vi "SetOIDNumbers.vi"(8 "error in (no error)":errorcluster, 11 "RoomAlert in":refnum<class "RoomAlert.lvclass">) -> (0 "error out":errorcluster, 3 "RoomAlert out":refnum<class "RoomAlert.lvclass">)   [LabVIEW 2018, in "SensorPlugins.lvlib" / "RoomAlert.lvclass"]
doc: "Sets the Sensor and the Light Tower OID Numbers that the operator may select from. The Module ID must be correct inorder for this function to work properly thus call GET&SET Instrument information before calling this VI."
uses:
  RoomAlert.lvclass
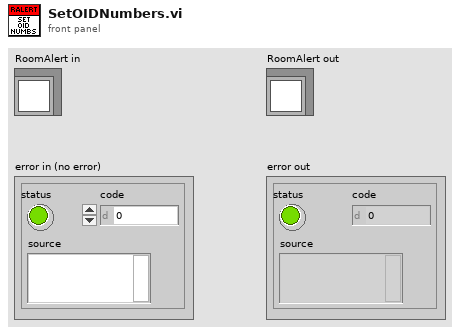
[diagram p1: front panel]
types:
  T1 = typedef "SensorPlugins.lvlib/RoomAlert.lvclass/RoomAlertControls.ctl" = cluster{"Connected?":bool, "IP Address of SNMP Device":string, "Port (161)":u16, "Community Name":string, "Measurements To Read Array":u16[], "Update LightTower?":bool, "LightTower":cluster{"Red":bool, "Amber":bool, "Green":bool, "Audio":bool}, "RoomAlert Model ID":string, "Sensor OID Numbers":string[][], "Sensor Light Tower OID Numbers":string[][]}[]
  T2 = cluster{"Connected?":bool, "IP Address of SNMP Device":string, "Port (161)":u16, "Community Name":string, "Measurements To Read Array":u16[], "Update LightTower?":bool, "LightTower":cluster{"Red":bool, "Amber":bool, "Green":bool, "Audio":bool}, "RoomAlert Model ID":string, "Sensor OID Numbers":string[][], "Sensor Light Tower OID Numbers":string[][]}
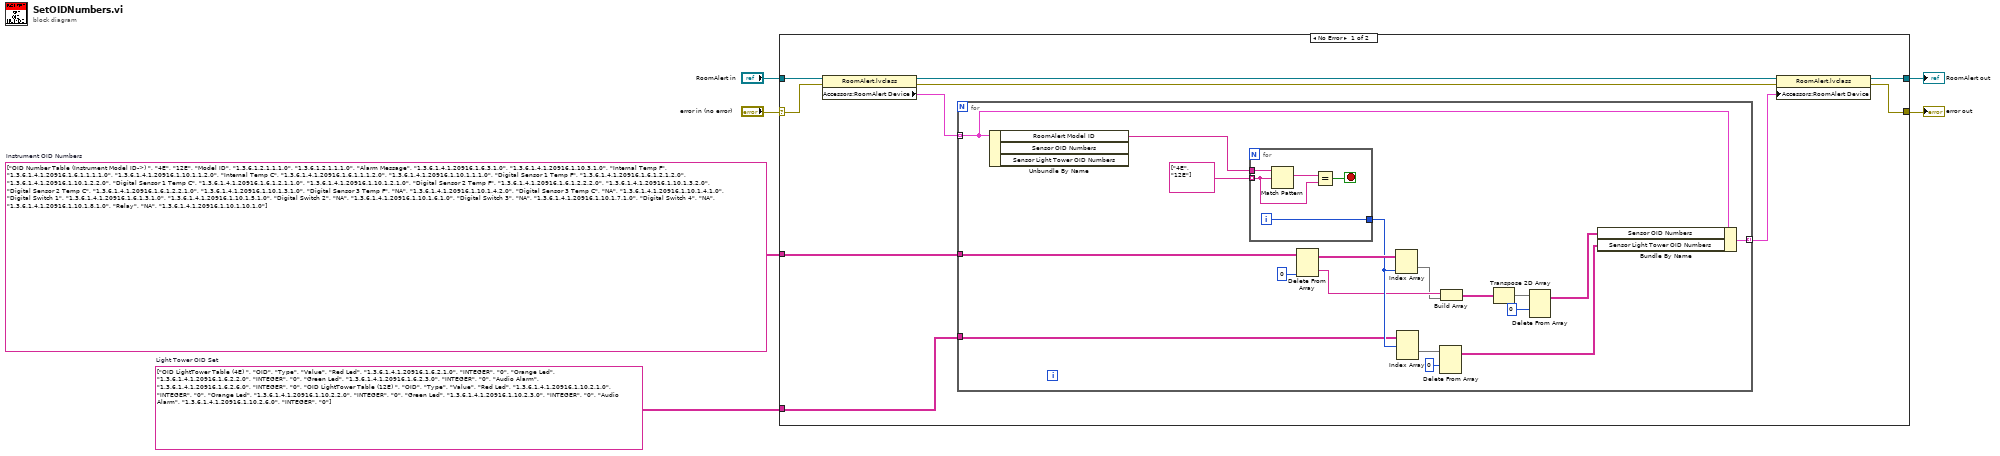
[diagram p0: block diagram]
diagram:
  w1 = string[][][] [[["OID LightTower Table (4E) ", "OID", "Type", "Value"], ["Red Led", "1.3.6.1.4.1.20916.1.6.2.1.0", "INTEGER", "0"], ["Orange Led", "1.3.6.1.4.1.20916.1.6.2.2.0", "INTEGER", "0"], ["Green Led", "1.3.6.1.4.1.20916.1.6.2.3.0", "INTEGER", "0"], ["Audio Alarm", "1.3.6.1.4.1.20916.1.6.2.6.0", "INTEGER", "0"]], [["OID LightTower Table (12E) ", "OID", "Type", "Value"], ["Red Led", "1.3.6.1.4.1.20916.1.10.2.1.0", "INTEGER", "0"], ["Orange Led", "1.3.6.1.4.1.20916.1.10.2.2.0", "INTEGER", "0"], ["Green Led", "1.3.6.1.4.1.20916.1.10.2.3.0", "INTEGER", "0"], ["Audio Alarm", "1.3.6.1.4.1.20916.1.10.2.6.0", "INTEGER", "0"]]]  # Light Tower OID Set
  w2 = string[][] [["OID Number Table (Instrument Model ID->) ", "4E", "12E"], ["Model ID", "1.3.6.1.2.1.1.1.0", "1.3.6.1.2.1.1.1.0"], ["Alarm Message", "1.3.6.1.4.1.20916.1.6.3.1.0", "1.3.6.1.4.1.20916.1.10.3.1.0"], ["Internal Temp F", "1.3.6.1.4.1.20916.1.6.1.1.1.1.0", "1.3.6.1.4.1.20916.1.10.1.1.2.0"], ["Internal Temp C", "1.3.6.1.4.1.20916.1.6.1.1.1.2.0", "1.3.6.1.4.1.20916.1.10.1.1.1.0"], ["Digital Sensor 1 Temp F", "1.3.6.1.4.1.20916.1.6.1.2.1.2.0", "1.3.6.1.4.1.20916.1.10.1.2.2.0"], ["Digital Sensor 1 Temp C", "1.3.6.1.4.1.20916.1.6.1.2.1.1.0", "1.3.6.1.4.1.20916.1.10.1.2.1.0"], ["Digital Sensor 2 Temp F", "1.3.6.1.4.1.20916.1.6.1.2.2.2.0", "1.3.6.1.4.1.20916.1.10.1.3.2.0"], ["Digital Sensor 2 Temp C", "1.3.6.1.4.1.20916.1.6.1.2.2.1.0", "1.3.6.1.4.1.20916.1.10.1.3.1.0"], ["Digital Sensor 3 Temp F", "NA", "1.3.6.1.4.1.20916.1.10.1.4.2.0"], ["Digital Sensor 3 Temp C", "NA", "1.3.6.1.4.1.20916.1.10.1.4.1.0"], ["Digital Switch 1", "1.3.6.1.4.1.20916.1.6.1.3.1.0", "1.3.6.1.4.1.20916.1.10.1.5.1.0"], ["Digital Switch 2", "NA", "1.3.6.1.4.1.20916.1.10.1.6.1.0"], ["Digital Switch 3", "NA", "1.3.6.1.4.1.20916.1.10.1.7.1.0"], ["Digital Switch 4", "NA", "1.3.6.1.4.1.20916.1.10.1.8.1.0"], ["Relay", "NA", "1.3.6.1.4.1.20916.1.10.1.10.1.0"]]  # Instrument OID Numbers
  n1 = case shown="No Error" "error in (no error)" {
    selector: "error in (no error)" -> [w14 w41]
    tunnel: [w12 w41] -> w5
    tunnel: [w11 w40] -> w3
    tunnel: "RoomAlert in" -> [w15 w40]
    tunnel: w2 -> [w8 _]
    tunnel: w1 -> [w7 _]
    frame No Error {
      n2 = property class="RoomAlert.lvclass"(reference=w15, error in=w14) -> (reference out=w10:refnum<class "RoomAlert.lvclass">, error out=w13:errorcluster, "Accessors:RoomAlert Device"=w16:T1)
      n3 = for {
        tunnel: w16 -> [w32] mode=indexing
        tunnel: [w31] -> w9 mode=indexing
        tunnel: w8 -> [w20]
        tunnel: w7 -> [w19]
        n4 = Unbundle By Name(w32) -> ("RoomAlert Model ID"=w33:string)  [unwired: 2 out]
        n5 = for {
          tunnel: w33 -> [w39]
          tunnel: string[] ["4E", "12E"] -> [w38] mode=indexing
          tunnel: [w35] -> w26
          i -> [w35]
          stop <- w36 stop-if-true
          n6 = Match Pattern(string=w39, regular expression=w38) -> (match substring=w37:string)  [unwired: 1 in, 3 out]
          n7 = Equal?(x=w37, y=w38) -> (x = y?=w36:bool)
        }
        n8 = Delete From Array(array=w20, index (col)=0 ("disabled index (col)")) -> (deleted portion=w24:string[], array with subset deleted=w27:string[][])  [unwired: 2 in]
        n9 = Index Array(array=w27, index (col)=w26) -> (element=w23:string[])  [unwired: 1 in]
        n10 = Index Array(array=w19, index (dim 0)=w26) -> (element=w30:string[][])  [unwired: 2 in]
        n11 = Delete From Array(array=w30, index (row)=0) -> (array with subset deleted=w17:string[][])  [unwired: 2 in, 1 out]
        n12 = Build Array(w24, w23) -> (w22:string[][])
        n13 = Transpose 2D Array(2D array=w22) -> (transposed array=w21:string[][])
        n14 = Delete From Array(array=w21, index (row)=0) -> (array with subset deleted=w18:string[][])  [unwired: 2 in, 1 out]
        n15 = Bundle By Name(cluster=w32, "Sensor OID Numbers"=w18, "Sensor Light Tower OID Numbers"=w17) -> (w31:T2)
      }
      n16 = property class="RoomAlert.lvclass"(reference=w10, error in=w13, "Accessors:RoomAlert Device"=w9) -> (reference out=w11:refnum<class "RoomAlert.lvclass">, error out=w12:errorcluster)
    }
    frame Error {
    }
  }
  "error out" <- w5
  "RoomAlert out" <- w3
